vi "wsFetchStates.vi"(8 "error in (no error)":errorcluster, 11 "References":T2) -> (0 "error out":errorcluster, 2 "states":T1(array[cluster]), 3 "Success?":bool)   [LabVIEW 2018, in "HASS-LV-WS_integration.lvlib"]
uses:
  HASS-LV-WS_integration.lvlib
  TypeDef/ReferencesTypeDef.ctl
  TypeDef/QueueTypeDef.ctl
  TypeDef/EventTypeDef.ctl
  <vilib>/addons/_JKI.lib/Serialization/JSON/JKI JSON Serialization.lvlib
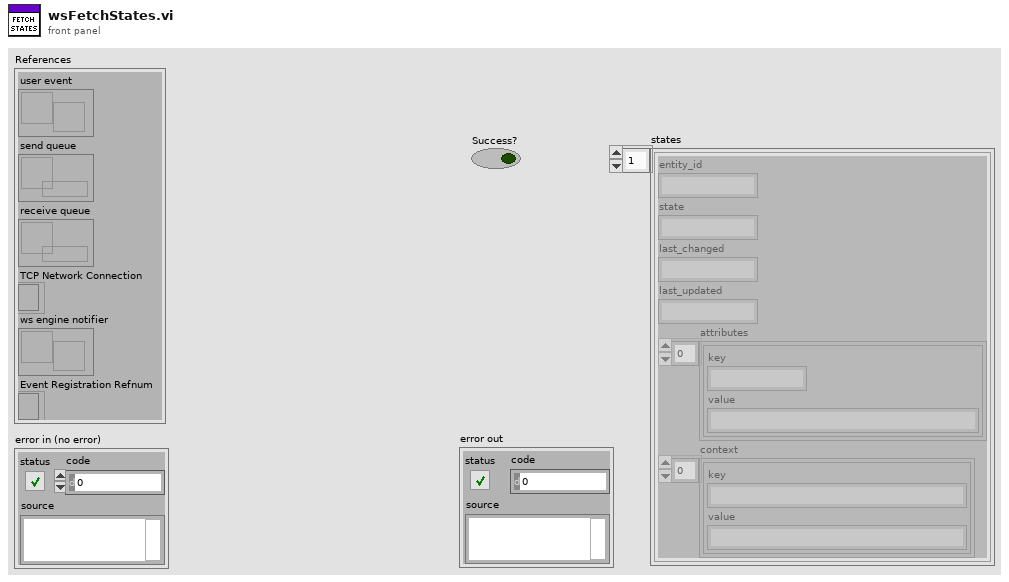
[diagram p1: front panel]
types:
  T1 = cluster{"entity_id":string, "state":string, "last_changed":string, "last_updated":string, "attributes":cluster{"key":string, "value":string}[], "context":cluster{"key":string, "value":string}[]}[]
  T2 = typedef "HASS-LV-WS_integration.lvlib/ReferencesTypeDef.ctl" = cluster{"user event":refnum<user-event>, "send queue":refnum<queue>, "receive queue":refnum<queue>, "TCP Network Connection":refnum<k5>, "ws engine notifier ":refnum<notifier>, "Event Registration Refnum":refnum<event-registration>}
  T3 = typedef "HASS-LV-WS_integration.lvlib/EventTypeDef.ctl" = cluster{"Data":variant, "Command":string}
  T4 = cluster{"entity_id":string, "state":string, "last_changed":string, "last_updated":string, "attributes":cluster{"key":string, "value":string}[], "context":cluster{"key":string, "value":string}[]}
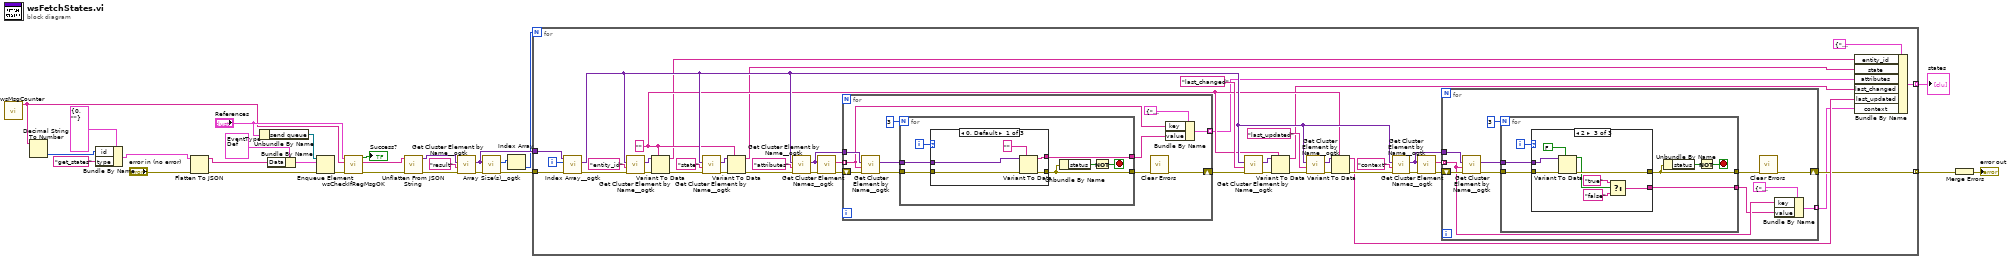
[diagram p0: block diagram]
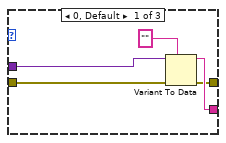
[diagram p2: hidden frame]
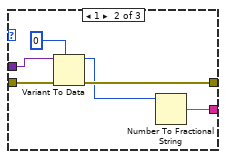
[diagram p3: hidden frame]
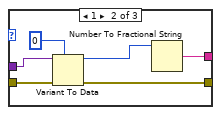
[diagram p4: hidden frame]
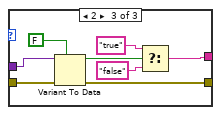
[diagram p5: hidden frame]
diagram:
  n1 = call "wsMsgCounter.vi"() -> ("msgCounter"=w25:string)  [unwired: 11 in]
  n2 = Decimal String To Number(string=w25) -> (number=w24:i32)  [unwired: 2 in, 1 out]
  n3 = Bundle By Name(cluster=cluster{"id":i32, "type":string} {"id"=0, "type"=""}, "id"=w24, "type"="get_states") -> (w17:cluster{"id":i32, "type":string})
  n4 = Flatten To JSON(anything=w17, error in (no error)="error in (no error)") -> (JSON string=w16:string, 11:w14:errorcluster)  [unwired: 1 in]
  n5 = Unbundle By Name("References") -> ("send queue"=w27:refnum<queue>)
  n6 = Bundle By Name(cluster=T3 {"Data"=variant, "Command"="Send"} ("element"), "Data"=w16) -> (w23:T3)
  n7 = Enqueue Element(queue=w27, element=w23, error in (no error)=w14) -> (error out=w22:errorcluster)  [unwired: 1 in, 2 out]
  n8 = call "wsCheckIfRegMsgOK.vi"("error in (no error)"=w22, "msgCounter"=w25, "References"="References") -> ("error out"=w13:errorcluster, "raw result"=w12:string, "Success?"=→"Success?":bool)  [unwired: 6 in]
  n9 = call <vilib>:"Unflatten From JSON String.vi"("error in (no error)"=w13, "JSON String"=w12) -> ("error out"=w5:errorcluster, "Variant"=w11:variant)  [unwired: 8 in]
  n10 = call <userlib>:"Get Cluster Element by Name__ogtk.vi"("error in (no error)"=w5, "Element Name"="result", "Cluster"=w11) -> ("error out"=w4:errorcluster, "VElement"=w9:variant)  [unwired: 6 in, 1 out]
  n11 = call <userlib>:"Array Size(s)__ogtk.vi"("error in (no error)"=w4, "Array"=w9) -> ("error out"=w3:errorcluster, "Size(s)"=w8:u32[])  [unwired: 7 in, 1 out]
  n12 = Index Array(array=w8) -> (element=w7:u32)  [unwired: 1 in]
  n13 = for {
    N: w7 -> [_]
    tunnel: w9 -> [w69]
    tunnel: [w41] -> w6 mode=indexing
    tunnel: [w31] -> w2 mode=indexing
    tunnel: w3 -> [w28]
    i -> [w68]
    w47 = ""
    n14 = call <userlib>:"Index Array__ogtk.vi"("error in (no error)"=w28, "Index (1D)"=w68, "MultiD Array"=w69) -> ("error out"=w61:errorcluster, "Array Element"=w60:variant)  [unwired: 7 in]
    n15 = call <userlib>:"Get Cluster Element by Name__ogtk.vi"("error in (no error)"=w61, "Element Name"="entity_id", "Cluster"=w60) -> ("error out"=w59:errorcluster, "VElement"=w51:variant)  [unwired: 6 in, 1 out]
    n16 = Variant To Data(error in=w59, type=w47, Variant=w51) -> (data=w45:string, error out=w58:errorcluster)
    n17 = call <userlib>:"Get Cluster Element by Name__ogtk.vi"("error in (no error)"=w58, "Element Name"="state", "Cluster"=w60) -> ("error out"=w57:errorcluster, "VElement"=w50:variant)  [unwired: 6 in, 1 out]
    n18 = Variant To Data(error in=w57, type=w47, Variant=w50) -> (data=w44:string, error out=w56:errorcluster)
    n19 = call <userlib>:"Get Cluster Element by Name__ogtk.vi"("error in (no error)"=w56, "Element Name"="attributes", "Cluster"=w60) -> ("error out"=w38:errorcluster, "VElement"=w40:variant)  [unwired: 6 in, 1 out]
    n20 = call <userlib>:"Get Cluster Element Names__ogtk.vi"("error in (no error)"=w38, "Cluster"=w40) -> ("error out"=w37:errorcluster, "Element Names"=w39:string[])  [unwired: 8 in]
    n21 = for {
      tunnel: w40 -> [w117]
      tunnel: w39 -> [w112] mode=indexing
      shift-right: [w107] -> w36
      shift-left: w37 -> [w114]
      tunnel: [w111] -> w35 mode=indexing
      n22 = call <userlib>:"Get Cluster Element by Name__ogtk.vi"("error in (no error)"=w114, "Element Name"=w112, "Cluster"=w117) -> ("error out"=w116:errorcluster, "VElement"=w109:variant)  [unwired: 6 in, 1 out]
      n23 = for {
        N: 3 -> [_]
        tunnel: [w123] -> w110
        tunnel: w109 -> [w122]
        tunnel: w116 -> [w124]
        tunnel: [w120] -> w115
        i -> [w121]
        stop <- w118 stop-if-true
        n24 = case shown="0, Default" w121 {
          tunnel: w124 -> [w125 w135 w143]
          tunnel: [w126 w132 w141] -> w120
          tunnel: [w127 w130 w137] -> w123
          tunnel: w122 -> [w128 w134 w142]
          frame 0, Default {
            n25 = Variant To Data(error in=w125, type="", Variant=w128) -> (data=w127:string, error out=w126:errorcluster)
          }
          frame 1 {
            n26 = Variant To Data(error in=w135, type=0, Variant=w134) -> (data=w131:i32, error out=w132:errorcluster)
            n27 = Number To Fractional String(number=w131) -> (F-format string=w130:string)  [unwired: 3 in]
          }
          frame 2 {
            n28 = Variant To Data(error in=w143, type=FALSE, Variant=w142) -> (data=w139:bool, error out=w141:errorcluster)
            n29 = Select(t="true", s=w139, f="false") -> (s? t:f=w137:string)
          }
        }
        n30 = Unbundle By Name(w120) -> ("status"=w119:bool)
        n31 = Not(x=w119) -> (.not. x?=w118:bool)
      }
      n32 = call <vilib>:"Clear Errors.vi"("error in (no error)"=w115) -> ("error out"=w107:errorcluster)  [unwired: 5 in, 1 out]
      n33 = Bundle By Name(cluster=cluster{"key":string, "value":string} {"key"="", "value"=""}, "key"=w112, "value"=w110) -> (w111:cluster{"key":string, "value":string})
    }
    n34 = call <userlib>:"Get Cluster Element by Name__ogtk.vi"("error in (no error)"=w36, "Element Name"="last_changed", "Cluster"=w60) -> ("error out"=w55:errorcluster, "VElement"=w49:variant)  [unwired: 6 in, 1 out]
    n35 = Variant To Data(error in=w55, type=w47, Variant=w49) -> (data=w43:string, error out=w54:errorcluster)
    n36 = call <userlib>:"Get Cluster Element by Name__ogtk.vi"("error in (no error)"=w54, "Element Name"="last_updated", "Cluster"=w60) -> ("error out"=w53:errorcluster, "VElement"=w48:variant)  [unwired: 6 in, 1 out]
    n37 = Variant To Data(error in=w53, type=w47, Variant=w48) -> (data=w42:string, error out=w52:errorcluster)
    n38 = call <userlib>:"Get Cluster Element by Name__ogtk.vi"("error in (no error)"=w52, "Element Name"="context", "Cluster"=w60) -> ("error out"=w34:errorcluster, "VElement"=w30:variant)  [unwired: 6 in, 1 out]
    n39 = call <userlib>:"Get Cluster Element Names__ogtk.vi"("error in (no error)"=w34, "Cluster"=w30) -> ("error out"=w33:errorcluster, "Element Names"=w32:string[])  [unwired: 8 in]
    n40 = for {
      tunnel: w30 -> [w80]
      tunnel: w32 -> [w77] mode=indexing
      shift-right: [w71] -> w31
      shift-left: w33 -> [w79]
      tunnel: [w76] -> w29 mode=indexing
      n41 = call <userlib>:"Get Cluster Element by Name__ogtk.vi"("error in (no error)"=w79, "Element Name"=w77, "Cluster"=w80) -> ("error out"=w75:errorcluster, "VElement"=w74:variant)  [unwired: 6 in, 1 out]
      n42 = for {
        N: 3 -> [_]
        tunnel: [w86] -> w72
        tunnel: w74 -> [w85]
        tunnel: w75 -> [w87]
        tunnel: [w83] -> w73
        i -> [w84]
        stop <- w81 stop-if-true
        n43 = case shown="2" w84 {
          tunnel: w87 -> [w88 w98 w106]
          tunnel: [w89 w95 w104] -> w83
          tunnel: [w90 w93 w100] -> w86
          tunnel: w85 -> [w91 w97 w105]
          frame 0, Default {
            n44 = Variant To Data(error in=w88, type="", Variant=w91) -> (data=w90:string, error out=w89:errorcluster)
          }
          frame 1 {
            n45 = Variant To Data(error in=w98, type=0, Variant=w97) -> (data=w94:i32, error out=w95:errorcluster)
            n46 = Number To Fractional String(number=w94) -> (F-format string=w93:string)  [unwired: 3 in]
          }
          frame 2 {
            n47 = Variant To Data(error in=w106, type=FALSE, Variant=w105) -> (data=w102:bool, error out=w104:errorcluster)
            n48 = Select(t="true", s=w102, f="false") -> (s? t:f=w100:string)
          }
        }
        n49 = Unbundle By Name(w83) -> ("status"=w82:bool)
        n50 = Not(x=w82) -> (.not. x?=w81:bool)
      }
      n51 = call <vilib>:"Clear Errors.vi"("error in (no error)"=w73) -> ("error out"=w71:errorcluster)  [unwired: 5 in, 1 out]
      n52 = Bundle By Name(cluster=cluster{"key":string, "value":string} {"key"="", "value"=""}, "key"=w77, "value"=w72) -> (w76:cluster{"key":string, "value":string})
    }
    n53 = Bundle By Name(cluster=T4 {"entity_id"="", "state"="", "last_changed"="", "last_updated"="", "attributes"=[], "context"=[]}, "entity_id"=w45, "state"=w44, "attributes"=w35, "last_changed"=w43, "last_updated"=w42, "context"=w29) -> (w41:T4)
  }
  "states" <- w6
  n54 = Merge Errors(w2) -> (→"error out":errorcluster)
